vi "TDC_setHistogramParams.vi"(8 "Error In":errorcluster, 10 "Bin Count":i32=2 min=2 max=1000000, 11 "Bin Width [native bins]":i32=1 min=1 max=1000000) -> (0 "Error Out":errorcluster)   [LabVIEW 2013]
uses:
  QUTAU-15_06_25/userlib/lib/tdcbase.dll
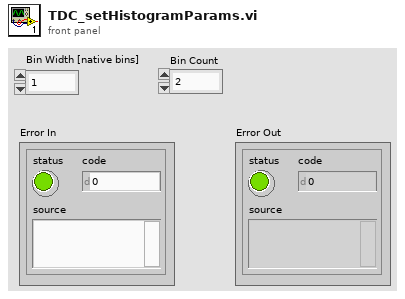
[diagram p1: front panel]
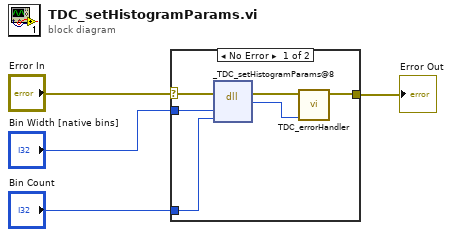
[diagram p0: block diagram]
diagram:
  n1 = case shown="No Error" "Error In" {
    selector: "Error In" -> [w8 w11]
    tunnel: [w5 w11] -> w4
    tunnel: "Bin Width [native bins]" -> [w10 _]
    tunnel: "Bin Count" -> [w9 _]
    frame No Error {
      n2 = dll-call lib="C:/Users/science/Desktop/NVExperimeent/Labview/QUTAU-15_06_25/userlib/lib/tdcbase.dll" fn="_TDC_setHistogramParams@8"(error in=w8, "binWidth"=w10, "binCount"=w9) -> (error out=w7:errorcluster, "return type"=w6:i32)  [unwired: 4 in, 1 out]
      n3 = call "TDC_errorHandler.vi"("quTAU Return Code"=w6, "Error In"=w7) -> ("Error Out"=w5:errorcluster)  [unwired: 9 in]
    }
    frame Error {
    }
  }
  "Error Out" <- w4
